vi "Get_Trigger.vi"(8 "error in (no error)":errorcluster, 11 "VISA resource name":refnum<visa-resource-name>="Master_Oscilloscope") -> (0 "error out":errorcluster, 2 "Trigger_Parameters":string[](array[string]), 3 "VISA resource name out":refnum<visa-resource-name>)   [LabVIEW 2020]
panel:
  out "Coupling":string
  out "Slope":string
  out "Level":string
  out "Source":string
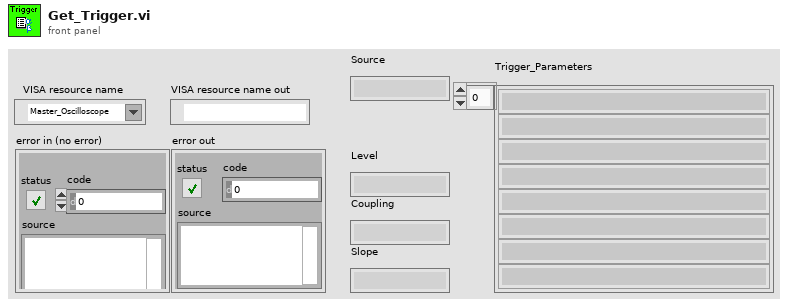
[diagram p1: front panel]
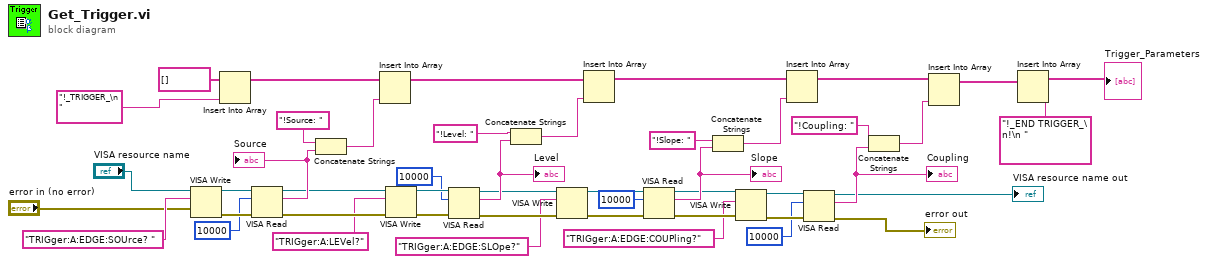
[diagram p0: block diagram]
diagram:
  n1 = VISA Write(VISA resource name="VISA resource name", write buffer="TRIGger:A:EDGE:SOUrce? ", error in (no error)="error in (no error)") -> (VISA resource name out=w46:refnum<visa-resource-name>, error out=w45:errorcluster)  [unwired: 1 out]
  n2 = Insert Into Array(array=string[] [], new element="!_TRIGGER_\n ") -> (w11:string[])  [unwired: 1 in]
  n3 = VISA Read(VISA resource name=w46, byte count=u32 10000, error in (no error)=w45) -> (VISA resource name out=w42:refnum<visa-resource-name>, read buffer=w44:string, error out=w41:errorcluster)  [unwired: 1 out]
  "Source" <- w44
  n4 = Concatenate Strings("!Source: " ("string"), w44) -> (w10:string)
  n5 = Insert Into Array(array=w11, new element=w10) -> (w9:string[])  [unwired: 1 in]
  n6 = VISA Write(VISA resource name=w42, write buffer="TRIGger:A:LEVel?", error in (no error)=w41) -> (VISA resource name out=w39:refnum<visa-resource-name>, error out=w38:errorcluster)  [unwired: 1 out]
  n7 = VISA Read(VISA resource name=w39, byte count=u32 10000, error in (no error)=w38) -> (VISA resource name out=w35:refnum<visa-resource-name>, read buffer=w37:string, error out=w34:errorcluster)  [unwired: 1 out]
  "Level" <- w37
  n8 = Concatenate Strings("!Level: " ("string"), w37) -> (w8:string)
  n9 = VISA Write(VISA resource name=w35, write buffer="TRIGger:A:EDGE:SLOpe?", error in (no error)=w34) -> (VISA resource name out=w32:refnum<visa-resource-name>, error out=w31:errorcluster)  [unwired: 1 out]
  n10 = Insert Into Array(array=w9, new element=w8) -> (w7:string[])  [unwired: 1 in]
  n11 = VISA Read(VISA resource name=w32, byte count=u32 10000, error in (no error)=w31) -> (VISA resource name out=w25:refnum<visa-resource-name>, read buffer=w27:string, error out=w24:errorcluster)  [unwired: 1 out]
  "Slope" <- w27
  n12 = Concatenate Strings("!Slope: ", w27) -> (w6:string)
  n13 = VISA Write(VISA resource name=w25, write buffer="TRIGger:A:EDGE:COUPling?", error in (no error)=w24) -> (VISA resource name out=w22:refnum<visa-resource-name>, error out=w21:errorcluster)  [unwired: 1 out]
  n14 = Insert Into Array(array=w7, new element=w6) -> (w5:string[])  [unwired: 1 in]
  n15 = VISA Read(VISA resource name=w22, byte count=u32 10000, error in (no error)=w21) -> (VISA resource name out=→"VISA resource name out":refnum<visa-resource-name>, read buffer=w19:string, error out=→"error out":errorcluster)  [unwired: 1 out]
  "Coupling" <- w19
  n16 = Concatenate Strings("!Coupling: ", w19) -> (w4:string)
  n17 = Insert Into Array(array=w5, new element=w4) -> (w3:string[])  [unwired: 1 in]
  n18 = Insert Into Array(array=w3, new element="!_END TRIGGER_\n!\n ") -> (→"Trigger_Parameters":string[])  [unwired: 1 in]
